vi "File Process VI.vi"(8 "error in (no error)":errorcluster, 11 "Parsed File Path":path) -> (0 "Error Out":errorcluster, 1 "Total Step":u64, 2 "Switching Times":u32[][](array[numeric]), 3 "Channel Names":string[](array[string]), 4 "Initial States":u16[](array[numeric]), 5 "Channel Number":u16, 6 "GPIB 1":string, 7 "GPIB 2":string)   [LabVIEW 2012]
panel:
  out "Time Step":dbl
  out "Total Time":dbl
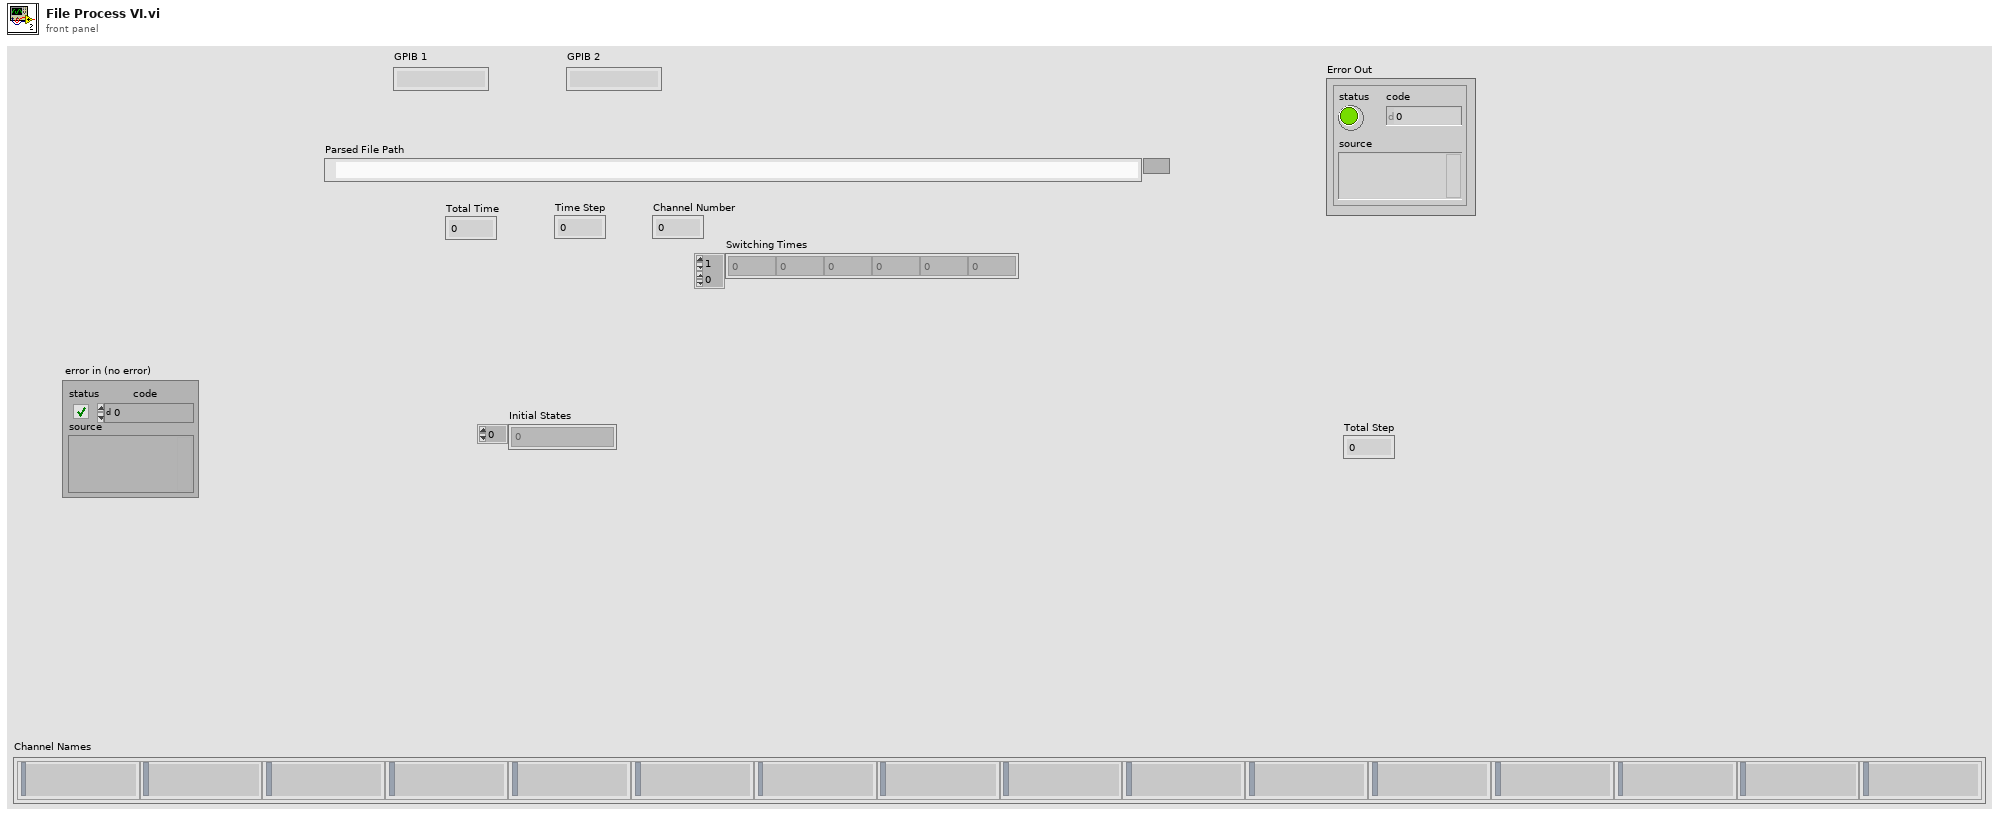
[diagram p1: front panel]
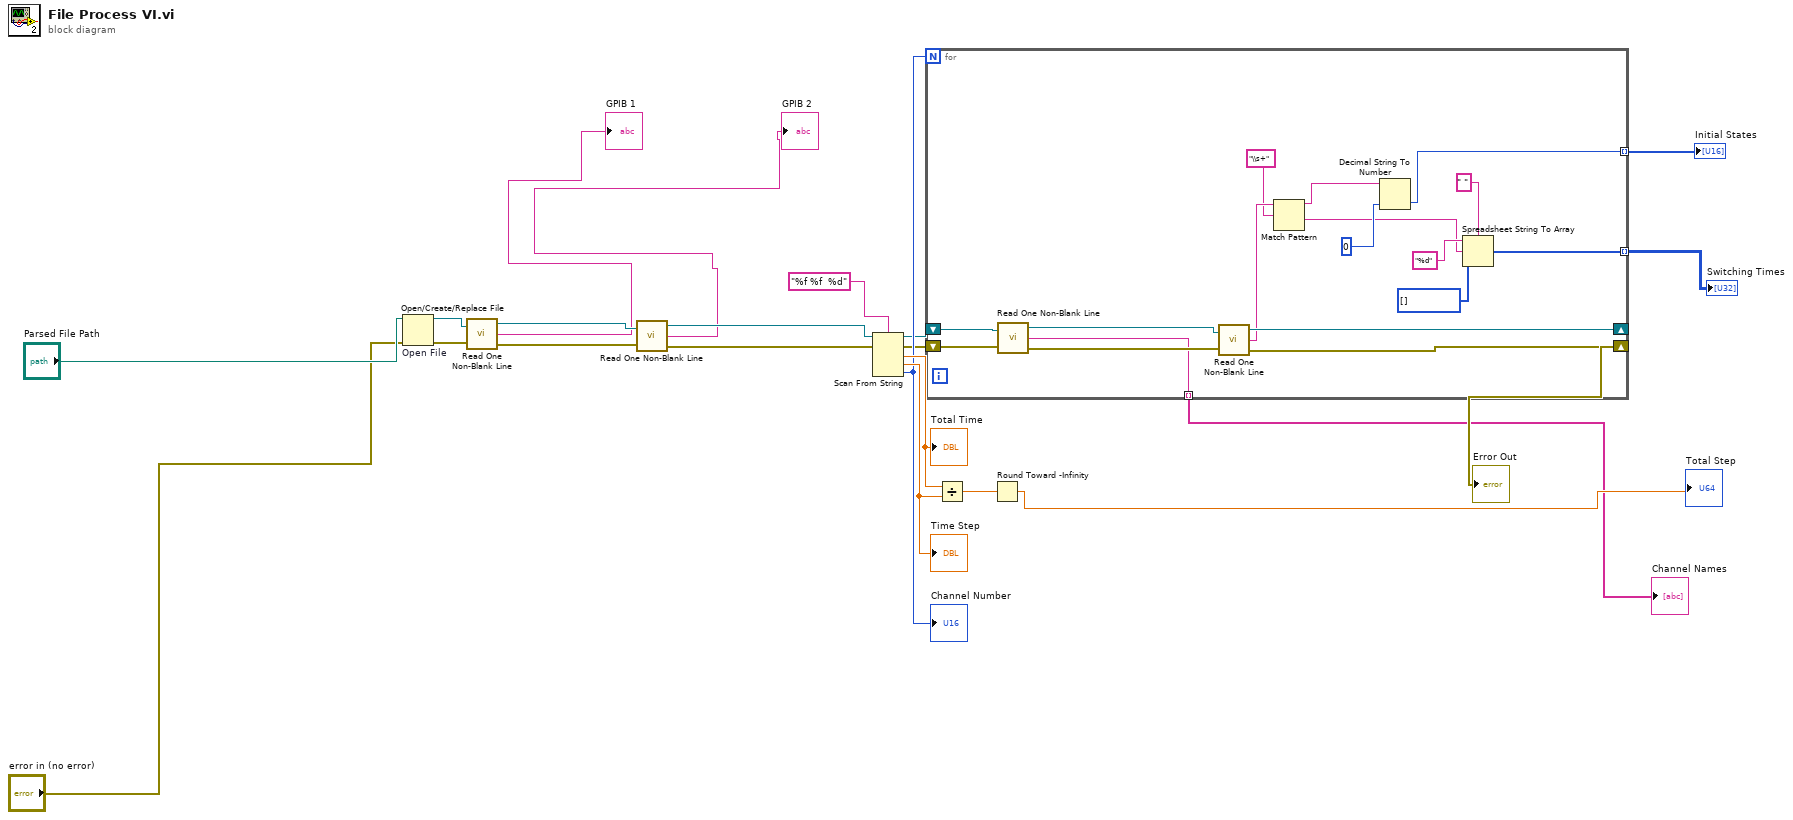
[diagram p0: block diagram]
diagram:
  n1 = Open/Create/Replace File "Open File"(file path (use dialog)="Parsed File Path", error in="error in (no error)") -> (refnum out=w21:refnum<file>, error out=w20:errorcluster)  [unwired: 4 in, 1 out]
  n2 = call "Read One Non-Blank Line.vi"("refnum"=w21, "error in (not an error)"=w20) -> ("dup refnum"=w19:refnum<file>, "Line"=→"GPIB 1":string, "error out"=w17:errorcluster)
  n3 = call "Read One Non-Blank Line.vi"("refnum"=w19, "error in (not an error)"=w17) -> ("dup refnum"=w18:refnum<file>, "Line"=→"GPIB 2":string, "error out"=w16:errorcluster)
  n4 = Scan From String("%f %f  %d", w18, w16) -> (w11:refnum<file>, w10:errorcluster, output 1=w15:dbl, output 2=w14:dbl, output 3=w12:u16)  [unwired: 3 in]
  "Total Time" <- w15
  "Time Step" <- w14
  "Channel Number" <- w12
  n5 = for {
    N: w12 -> [_]
    shift-right: [w37] -> _
    shift-left: w11 -> [w39]
    shift-right: [w34] -> w8
    shift-left: w10 -> [w36]
    tunnel: [w33] -> w6 mode=indexing
    tunnel: [w24] -> w9 mode=indexing
    tunnel: [w23] -> w5 mode=indexing
    n6 = call "Read One Non-Blank Line.vi"("refnum"=w39, "error in (not an error)"=w36) -> ("dup refnum"=w38:refnum<file>, "Line"=w33:string, "error out"=w35:errorcluster)
    n7 = call "Read One Non-Blank Line.vi"("refnum"=w38, "error in (not an error)"=w35) -> ("dup refnum"=w37:refnum<file>, "Line"=w32:string, "error out"=w34:errorcluster)
    n8 = Match Pattern(string=w32, regular expression="\\s+" ("search char (-)")) -> (before substring=w27:string, after substring=w25:string)  [unwired: 1 in, 2 out]
    n9 = Decimal String To Number(string=w27, default (0L)=u16 0) -> (number=w24:u16)  [unwired: 1 in, 1 out]
    n10 = Spreadsheet String To Array(delimiter (Tab)=" ", format string="%d", spreadsheet string=w25, array type (2D Dbl)=u32[] []) -> (array=w23:u32[])
  }
  "Switching Times" <- w5
  "Initial States" <- w9
  "Error Out" <- w8
  "Channel Names" <- w6
  n11 = Divide(x=w15, y=w14) -> (x/y=w13:dbl)
  n12 = Round Toward -Infinity(1:w13) -> (0:→"Total Step":dbl)
